vi "close.vi"(8 "error in":errorcluster, 11 "Tag Bus Web Interface runtime in":refnum<class "Tag Bus Web Interface runtime.lvclass">) -> (0 "error out":errorcluster)   [LabVIEW 2013, in "Tag Bus Web Interface runtime.lvclass"]
doc: "Provides an interface for terminating a module instance. While this interface performs no operations, a child should close and deallocate any open references or memory."
uses:
  Tag Bus Web Interface runtime.lvclass
  Tag Bus Web Interface runtime.lvclass/Tag Bus Web Interface runtime.ctl
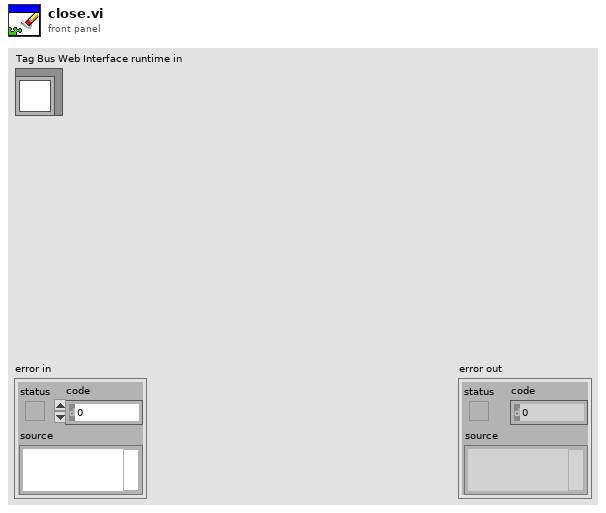
[diagram p1: front panel]
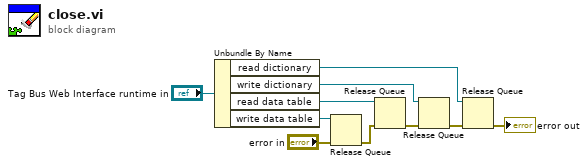
[diagram p0: block diagram]
diagram:
  n1 = Unbundle By Name("Tag Bus Web Interface runtime in") -> ("read dictionary"=w4:refnum<queue>, "write dictionary"=w3:refnum<queue>, "read data table"=w2:refnum<queue>, "write data table"=w1:refnum<queue>)
  n2 = Release Queue(queue=w1, error in (no error)="error in") -> (error out=w8:errorcluster)  [unwired: 1 in, 2 out]
  n3 = Release Queue(queue=w2, error in (no error)=w8) -> (error out=w9:errorcluster)  [unwired: 1 in, 2 out]
  n4 = Release Queue(queue=w3, error in (no error)=w9) -> (error out=w5:errorcluster)  [unwired: 1 in, 2 out]
  n5 = Release Queue(queue=w4, error in (no error)=w5) -> (error out=→"error out":errorcluster)  [unwired: 1 in, 2 out]
